vi "saveLogEntry.vi"(8 "error in (no error)":errorcluster, 11 "Logger in":refnum<class "LoggerDatalog.lvclass">) -> (0 "error out":errorcluster, 3 "Logger out":refnum<class "LoggerDatalog.lvclass">)   [LabVIEW 2013, in "LoggerDatalog.lvclass"]
uses:
  LoggerDatalog.lvclass
  Typedefs/LogRecord.ctl
  Typedefs/InputData.ctl
  <userlib>/Common/ILC/Typedefs/LimitSwitches.ctl
  Typedefs/ForceDemand.ctl
  Typedefs/Distance Data.ctl
  Typedefs/TemperatureData.ctl
  Typedefs/ControllerData.ctl
  Typedefs/OutputData.ctl
  Typedefs/StateSelector.ctl
  LoggerDatalog.lvclass/LoggerDatalog.ctl
  <userlib>/Common/ILC/Typedefs/ILCTypedefs.lvlib
  Typedefs/M2AADTTypedefs.lvlib
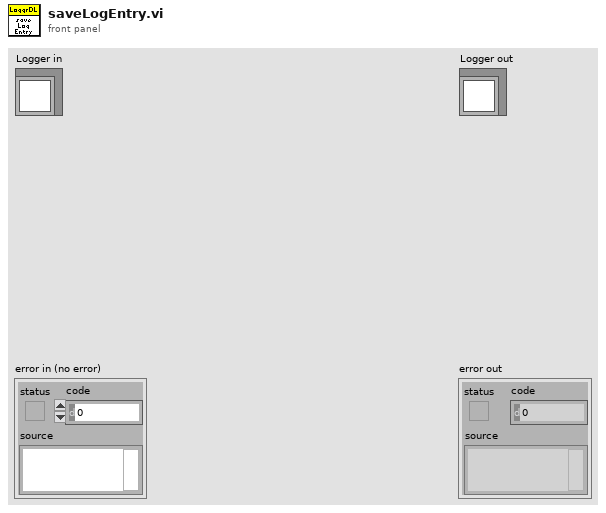
[diagram p1: front panel]
types:
  T1 = typedef "M2AADTTypedefs.lvlib/LogRecord.ctl" = cluster{"Time Stamp":timestamp, "Input Data":T2, "Controller Data":T7, "Output Data":T8, "State:":T9}
  T2 = typedef "M2AADTTypedefs.lvlib/InputData.ctl" = cluster{"Limit Switches":T3, "SSI Encoder":i32, "Force Measured":T4, "Distance Data":T5, "Temperature Data":T6}
  T3 = typedef "ILCCommon.lvlib/ILCTypedefs.lvlib/LimitSwitches.ctl" = cluster{"1":bool, "2":bool}
  T4 = typedef "M2AADTTypedefs.lvlib/ForceDemand.ctl" = dbl[unit]
  T5 = typedef "M2AADTTypedefs.lvlib/Distance Data.ctl" = cluster{"Distance Measured 1":dbl[unit], "Distance Measured 2":dbl[unit]}
  T6 = typedef "M2AADTTypedefs.lvlib/TemperatureData.ctl" = cluster{"Ambient Temperature":dbl[unit], "Motor Temperature":dbl[unit]}
  T7 = typedef "M2AADTTypedefs.lvlib/ControllerData.ctl" = cluster{"Force Demand":T4, "Force Error":T4}
  T8 = typedef "M2AADTTypedefs.lvlib/OutputData.ctl" = cluster{"Step & Direction":i16}
  T9 = typedef "M2AADTTypedefs.lvlib/StateSelector.ctl" = enum16{"EndingCycleState", "FaultState", "InteractiveMotionState", "MovingToNewForceState", "OffState", "PausingState", "StandbyState", "StoppedState"}
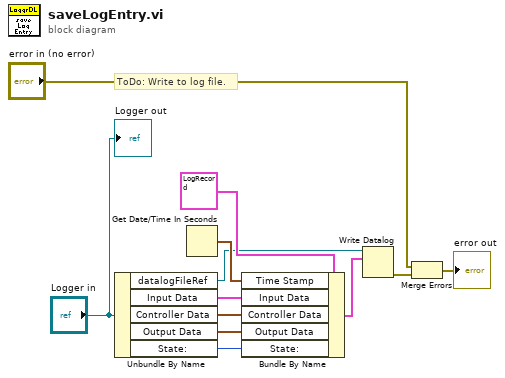
[diagram p0: block diagram]
diagram:
  # "ToDo: Write to log file."
  n1 = Unbundle By Name("Logger in") -> ("datalogFileRef"=w8:refnum<k1>, "Input Data"=w7:T2, "Controller Data"=w6:T7, "Output Data"=w5:T8, "State:"=w4:T9)
  n2 = Get Date/Time In Seconds() -> (seconds since 1Jan1904=w10:timestamp)
  n3 = Bundle By Name(cluster=T1 {"Time Stamp"=timestamp(0 s since 1904-01-01), "Input Data"={"Limit Switches"={"1"=FALSE, "2"=FALSE}, "SSI Encoder"=0, "Force Measured"=0.0, "Distance Data"={"Distance Measured 1"=1.0, "Distance Measured 2"=1.0}, "Temperature Data"={"Ambient Temperature"=274.15, "Motor Temperature"=274.15}}, "Controller Data"={"Force Demand"=0.0, "Force Error"=0.0}, "Output Data"={"Step & Direction"=0}, "State:"=enum."EndingCycleState"} ("Log Record"), "Time Stamp"=w10, "Input Data"=w7, "Controller Data"=w6, "Output Data"=w5, "State:"=w4) -> (w9:T1)
  n4 = Write Datalog(6:w9, 7:w8) -> (0:w2:errorcluster)  [unwired: 1 in, 1 out]
  n5 = Merge Errors("error in (no error)", w2) -> (→"error out":errorcluster)
  "Logger out" <- "Logger in"
